vi "Clear Error Code.vi"(8 "error in (no error)":errorcluster, 11 "Code":i32) -> (0 "error out":errorcluster)   [LabVIEW 2020, in "Engine Simulation Toolkit Engine.lvlib"]
uses:
  Engine Simulation Toolkit Engine.lvlib
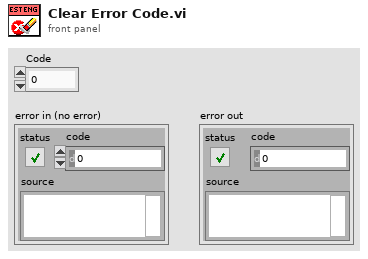
[diagram p1: front panel]
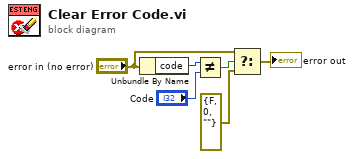
[diagram p0: block diagram]
diagram:
  n1 = Unbundle By Name("error in (no error)") -> ("code"=w1:i32)
  n2 = Not Equal?(x=w1, y="Code") -> (x != y?=w3:bool)
  n3 = Select(t="error in (no error)", s=w3, f=errorcluster {"status"=FALSE, "code"=0, "source"=""}) -> (s? t:f=→"error out":errorcluster)
